vi "Read Control Label.vi"(8 "error in (no error)":errorcluster, 11 "ControlMouseEnterMsg in":refnum<class "ControlMouseEnterMsg.lvclass">) -> (0 "error out":errorcluster, 2 "Control Label":string, 3 "ControlMouseEnterMsg out":refnum<class "ControlMouseEnterMsg.lvclass">)   [LabVIEW 2017, in "ActorEvents.lvlib" / "ControlMouseEnterMsg.lvclass"]
uses:
  ControlMouseEnterMsg.lvclass
  ControlMouseEnterMsg.lvclass/ControlMouseEnterMsg.ctl
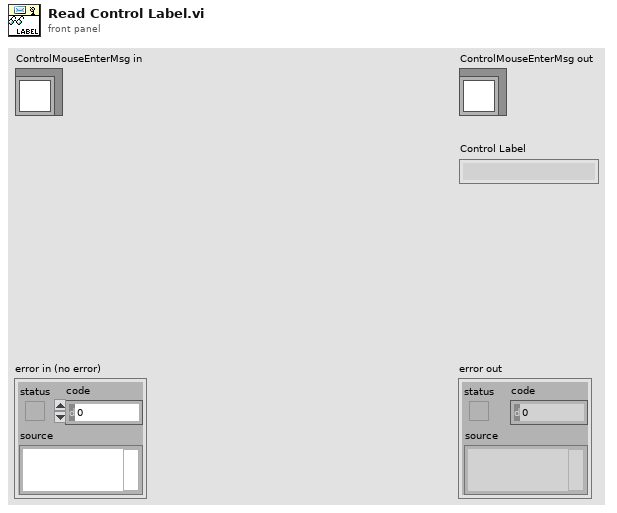
[diagram p1: front panel]
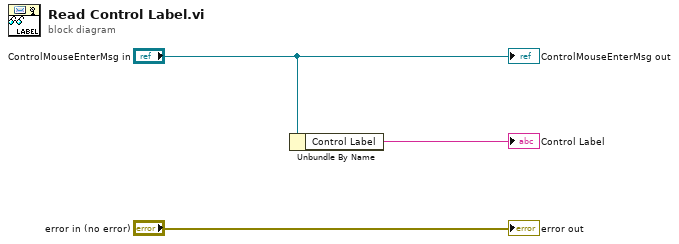
[diagram p0: block diagram]
diagram:
  n1 = Unbundle By Name("ControlMouseEnterMsg in") -> ("Control Label"=→"Control Label":string)
  "error out" <- "error in (no error)"
  "ControlMouseEnterMsg out" <- "ControlMouseEnterMsg in"
